vi "MARS_Scan_Global_var.vi"() -> ()   [LabVIEW 2015]
uses:
  <vilib>/Analysis/6fits.llb/Curve Fitting Criteria.ctl
  <vilib>/Analysis/NI_AALPro.lvlib
panel:
  in  "Fit method":T1=2 items=["Least Square", "Least Absolute Residual", "Bisquare"]
  in  "Fit std":dbl=1.0 format="%#_13g"
  in  "Fit index":i32=1
  in  "Fit thr":dbl=10.0 format="%#_13g"
  in  "Fit width":i32=5
  in  "Nb of Steps 2":u16 caption="Nb of Steps" step=1
  in  "Step 2":dbl caption="Step Size (us)" min=0.0 max=10.0 step=0.0208 format="%#.3g"
  in  "Int. per. 2":dbl caption="First Value (us)" min=0.0 max=9.0 step=0.0208 format="%#.3g"
  in  "Nb of Steps 1":u16 caption="Nb of Steps" step=1
  in  "Step 1":dbl caption="Step Size (us)" min=0.0 max=10.0 step=0.0208 format="%^#.3g"
  in  "Int. per. 1":dbl caption="First Value (us)" min=0.0 max=8.0 step=0.0208 format="%#.3g"
  in  "Nb of Frames":u32=400 min=100 step=100
  # "1st Integr. Period\n Scan Values"
  # "2nd Integr. Period\n Scan Values"
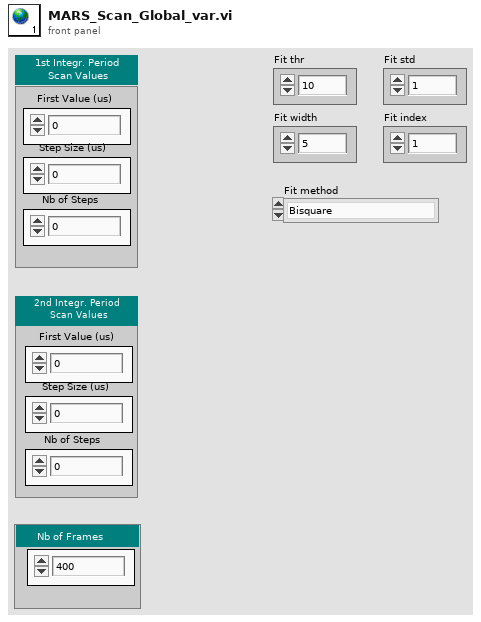
[diagram p1: front panel]
types:
  T1 = typedef "NI_AALPro.lvlib/Curve Fitting Criteria.ctl" = u16
diagram:
